vi "Test Write Data.vi"() -> ()   [LabVIEW 2014]
uses:
  ALPHA5 RS485/typedefs/Port Selection Info.ctl
  ALPHA5 RS485/ALPHA5 RS485.lvlib
panel:
  in  "Specified Num in":u8=1
  out "CRC Match":bool
  out "error out":errorcluster
  in  "Address":u16=65535 format="%.0x"
  in  "Data":i32[](array[numeric])
  in  "error in (no error)":errorcluster caption="error in（no error）"
  in  "Port Selection Info In":T1={"Port Name"="COM5", "Amplifier Num"=1, "Baud Rate"=38400, "Char Formation"=enum."0"} {"Baud Rate" items=["38400"=38400, "19200"=19200, "9600"=9600, "115200"=0]; "Amplifier Num" max=31}
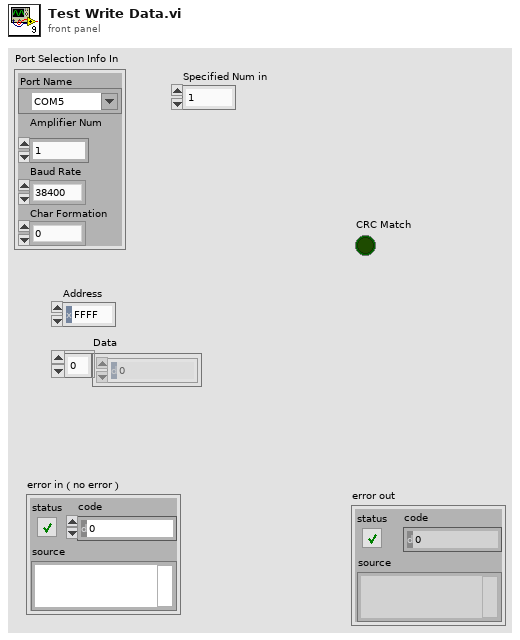
[diagram p1: front panel]
types:
  T1 = typedef "ALPHA5 RS485.lvlib/Port Selection Info.ctl" = cluster{"Port Name":refnum<visa-resource-name>, "Amplifier Num":u8, "Baud Rate":u32, "Char Formation":enum16{"0", "1", "2", "3", "4", "5"}}
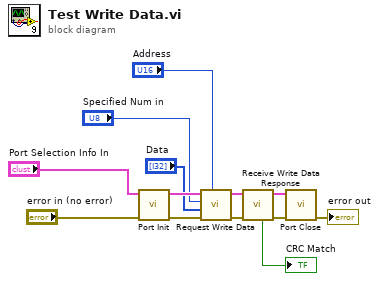
[diagram p0: block diagram]
diagram:
  n1 = call "Port Init.vi"("error in (no error)"="error in (no error)", "Port Selection Info In"="Port Selection Info In") -> ("error out"=w10:errorcluster, "Port Selection Info Out"=w12:T1)  [unwired: 8 in]
  n2 = call "Request Write Data.vi"("Address"="Address", "error in (no error)"=w10, "Data"="Data", "Specified Num in"="Specified Num in", "Port Selection Info"=w12) -> ("error out"=w6:errorcluster, "Port Selection Info Out"=w7:T1)  [unwired: 4 in, 1 out]
  n3 = call "Receive Write Data Response.vi"("error in (no error)"=w6, "Port Selection Info"=w7) -> ("error out"=w4:errorcluster, "Port Selection Info Out"=w5:T1, "CRC Match"=→"CRC Match":bool)  [unwired: 3 in, 4 out]
  n4 = call "Port Close.vi"("error in (no error)"=w4, "Port Selection Info In"=w5) -> ("error out"=→"error out":errorcluster)  [unwired: 9 in]
